vi "FT_Open_Device_By_Description.vi"(8 "error in":errorcluster, 11 "Device Description":string) -> (0 "error out":errorcluster, 3 "Handle":u32)   [LabVIEW 2016]
uses:
  FTD2XX.dll
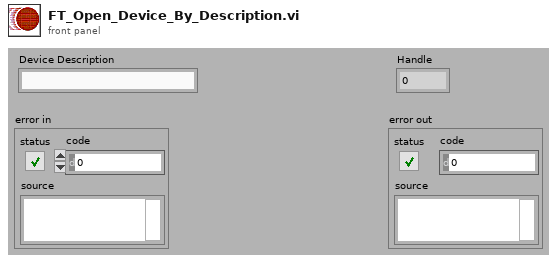
[diagram p1: front panel]
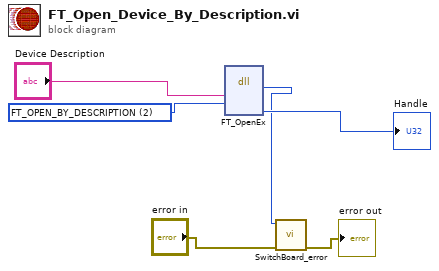
[diagram p0: block diagram]
diagram:
  w4 = u32 2 items=["FT_OPEN_BY_SERIAL_NUMBER"=1, "FT_OPEN_BY_DESCRIPTION"=2, "FT_OPEN_BY_LOCATION"=4] ("Flags")
  n1 = dll-call lib="FTD2XX.dll" fn="FT_OpenEx"("DeviceDescription"="Device Description", "Flags"=w4) -> ("FT_Status"=w1:u32, "Handle"=→"Handle":u32)  [unwired: 6 in, 2 out]
  n2 = call "SwitchBoard_error.vi"("error constant"="error in", "Code"=w1) -> ("error IO"=→"error out":errorcluster)  [unwired: 9 in]
